vi "获取最新一笔数据.vi"(8 "error in (no error)":errorcluster caption="错误输入（无错误）", 10 "table":string, 11 "database":string) -> (0 "error out":errorcluster caption="错误输出", 3 "子数组":variant[](array[variant]))   [LabVIEW 2016, in "database.lvlib"]
uses:
  database.lvlib
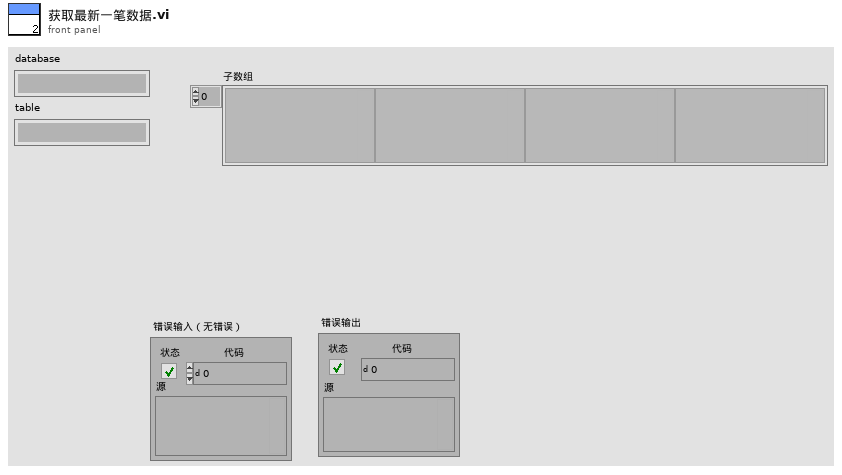
[diagram p1: front panel]
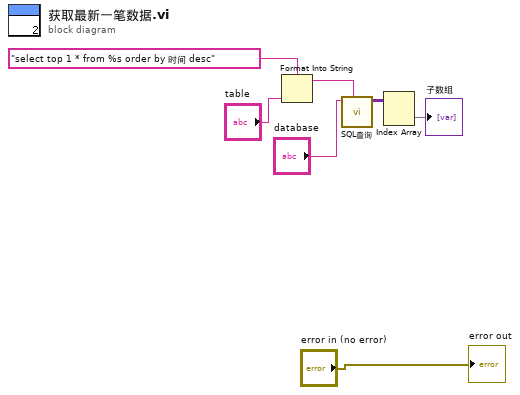
[diagram p0: block diagram]
diagram:
  n1 = Format Into String(format string="select top 1 * from %s order by 时间 desc" ("格式字符串"), "table") -> (resulting string=w6:string)  [unwired: 2 in, 1 out]
  n2 = call "SQL查询.vi"("SQL query"=w6, "database"="database") -> ("recordset data"=w3:variant[][])  [unwired: 8 in, 1 out]
  n3 = Index Array(array=w3) -> (element=→"子数组":variant[])  [unwired: 2 in]
  "error out" <- "error in (no error)"
